vi "MonitorOperationOnCluster.vi"(6 "YScale.Range":T2, 9 "Plot Area Size":T1, 10 "Original Zoom rect coords":T3, 11 "XScale.Range":T2) -> (3 "Rect coords  graph scale":T4)   [LabVIEW 2016]
uses:
  <vilib>/Utility/miscctls.llb/LVRangeTypeDef.ctl
  <vilib>/Utility/miscctls.llb/LVBoundsTypeDef.ctl
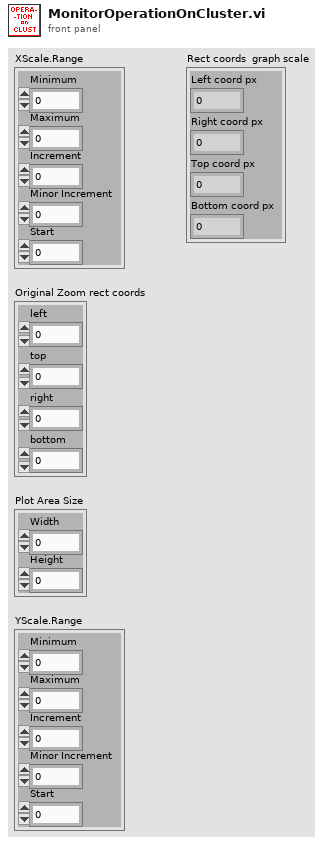
[diagram p1: front panel]
types:
  T1 = typedef "LVBoundsTypeDef.ctl" = cluster{"Width":u32, "Height":u32}
  T2 = typedef "LVRangeTypeDef.ctl" = cluster{"Minimum":dbl, "Maximum":dbl, "Increment":dbl, "Minor Increment":dbl, "Start":dbl}
  T3 = cluster{"left":i16, "top":i16, "right":i16, "bottom":i16}
  T4 = cluster{"Left coord px":dbl, "Right coord px":dbl, "Top coord px":dbl, "Bottom coord px":dbl}
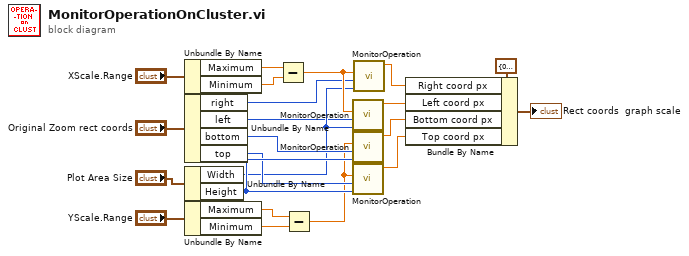
[diagram p0: block diagram]
diagram:
  n1 = Unbundle By Name("XScale.Range") -> ("Maximum"=w6:dbl, "Minimum"=w5:dbl)
  n2 = Unbundle By Name("Original Zoom rect coords") -> ("right"=w10:i16, "left"=w11:i16, "bottom"=w15:i16, "top"=w17:i16)
  n3 = Unbundle By Name("Plot Area Size") -> ("Width"=w12:u32, "Height"=w18:u32)
  n4 = Unbundle By Name("YScale.Range") -> ("Maximum"=w3:dbl, "Minimum"=w2:dbl)
  n5 = Subtract(x=w6, y=w5) -> (x-y=w13:dbl)
  n6 = Subtract(x=w3, y=w2) -> (x-y=w14:dbl)
  n7 = call "MonitorOperation.vi"("Width"=w12, "Right"=w11, "Max - Min"=w13) -> ("Conversion"=w20:dbl)  [unwired: 8 in]
  n8 = call "MonitorOperation.vi"("Width"=w18, "Right"=w15, "Max - Min"=w14) -> ("Conversion"=w16:dbl)  [unwired: 8 in]
  n9 = call "MonitorOperation.vi"("Width"=w18, "Right"=w17, "Max - Min"=w14) -> ("Conversion"=w22:dbl)  [unwired: 8 in]
  n10 = call "MonitorOperation.vi"("Width"=w12, "Right"=w10, "Max - Min"=w13) -> ("Conversion"=w21:dbl)  [unwired: 8 in]
  n11 = Bundle By Name(cluster=T4 {"Left coord px"=0.0, "Right coord px"=0.0, "Top coord px"=0.0, "Bottom coord px"=0.0} ("Rect coords  graph scale"), "Right coord px"=w21, "Left coord px"=w20, "Bottom coord px"=w16, "Top coord px"=w22) -> (→"Rect coords  graph scale":T4)
